vi "测试.vi"() -> ()   [LabVIEW 2016, in "WL-1A1.lvlib"]
uses:
  WL-1A1.lvlib
  <vilib>/Plasmionique/MB Master/MB_Master_Serial/MB_Master_Serial.lvclass
  D:/Program Files (x86)/National Instruments/LabVIEW 2016/vi.lib/Plasmionique/MB Master/MB_Master/MB_Master.lvclass
panel:
  out "读取值":cluster{"瞬时流量":dbl, "累计流量":dbl, "水位":dbl}
  in  "功能输入":enum16{"打开串口", "关闭串口"}(ring)
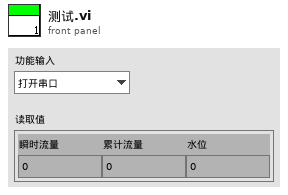
[diagram p1: front panel]
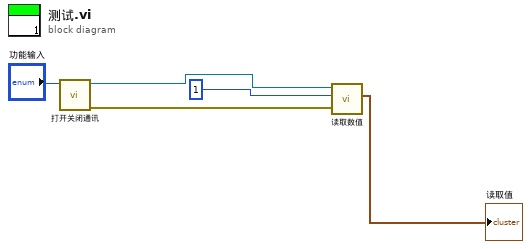
[diagram p0: block diagram]
diagram:
  n1 = call "打开关闭通讯.vi"("功能输入"="功能输入") -> ("error out"=w5:errorcluster, "MB_Serial session"=w3:refnum<class "MB_Master_Serial.lvclass">)  [unwired: 9 in]
  n2 = call "读取数值.vi"("error in (no error)"=w5, "Slave ID"=u8 1, "MB session in"=w3) -> ("读取值"=→"读取值":cluster{"瞬时流量":sgl, "累计流量":sgl, "水位":sgl})  [unwired: 6 in, 2 out]
